vi "rsscope_core_global.vi"() -> ()   [LabVIEW 2014] (continued)
"Data Type"=0, "Command"="SEAR:TRIG:DPHY:ESDT:COND", "Access"=2, "Range Table"="rsscope_rngProtocolTriggerCondition", "Read Callback"="rsscope_FormatSearchNameInt32_ReadCallback.vi", "Write Callback"="rsscope_FormatSearchNameInt32_WriteCallback.vi", "Supported Models"="", "Instrument Options"="K42", "Flags"=0, "Help"="Set the condition for the escape mode data value. You can define an exact value or a value range.\n\nAvailable Repeated Capabilities:\nNone\n\nRemote-control command(s):\nSEARch:TRIGger:DPHY:ESDTa:CONDition"}, {"Level"=5, "Class Only"=FALSE, "Identifier"="RSSCOPE_ATTR_DPHY_SEARCH_LOW_POWER_ESCAPE_MODE_DATA_MIN", "Descriptive Name"="DPHY Search Low Power Escape Mode Data Min", "Data Type"=2, "Command"="SEAR:TRIG:DPHY:ESDT:MIN", "Access"=2, "Range Table"="", "Read Callback"="rsscope_FormatSearchNameString_ReadCallback.vi", "Write Callback"="rsscope_FormatSearchNameString_WriteCallback.vi", "Supported Models"="", "Instrument Options"="K42", "Flags"=0, "Help"="Specifies an escape mode data bit pattern, or sets the start value of a pattern range.\n\nValid Values:\nBinary pattern string consisting of 1; 0; or X (any bit).\n\nAvailable Repeated Capabilities:\nNone\n\nRemote-control command(s):\nSEARch:TRIGger:DPHY:ESDTa:MIN"}, {"Level"=5, "Class Only"=FALSE, "Identifier"="RSSCOPE_ATTR_DPHY_SEARCH_LOW_POWER_ESCAPE_MODE_DATA_MAX", "Descriptive Name"="DPHY Search Low Power Escape Mode Data Max", "Data Type"=2, "Command"="SEAR:TRIG:DPHY:ESDT:MAX", "Access"=2, "Range Table"="", "Read Callback"="rsscope_FormatSearchNameString_ReadCallback.vi", "Write Callback"="rsscope_FormatSearchNameString_WriteCallback.vi", "Supported Models"="", "Instrument Options"="K42", "Flags"=0, "Help"="Sets the end value of a escape mode data type range for condition In Range or Out of Range. \n\nValid Values:\nBinary pattern string consisting of 1; 0; or X (any bit).\n\nAvailable Repeated Capabilities:\nNone\n\nRemote-control command(s):\nSEARch:TRIGger:DPHY:ESDTa:MAX"}, {"Level"=4, "Class Only"=TRUE, "Identifier"="", "Descriptive Name"="Data Index", "Data Type"=0, "Command"="", "Access"=0, "Range Table"="", "Read Callback"="", "Write Callback"="", "Supported Models"="", "Instrument Options"="", "Flags"=0, "Help"="Data index sets the range within this series of the data value that is considered for the analysis. The data index setup consists of the condition and one or two data index values."}, {"Level"=5, "Class Only"=FALSE, "Identifier"="RSSCOPE_ATTR_DPHY_SEARCH_HIGH_SPEED_DATA_INDEX_CONDITION", "Descriptive Name"="DPHY Search High Speed Data Index Condition", "Data Type"=0, "Command"="SEAR:TRIG:DPHY:DIDX:COND", "Access"=2, "Range Table"="rsscope_rngProtocolTriggerCondition", "Read Callback"="rsscope_FormatSearchNameInt32_ReadCallback.vi", "Write Callback"="rsscope_FormatSearchNameInt32_WriteCallback.vi", "Supported Models"="", "Instrument Options"="K42", "Flags"=0, "Help"="Sets the condition for the data index. You can define an exact value or a value range.\n\nAvailable Repeated Capabilities:\nNone\n\nRemote-control command(s):\nSEARch:TRIGger:DPHY:DIDX:CONDition"}, {"Level"=5, "Class Only"=FALSE, "Identifier"="RSSCOPE_ATTR_DPHY_SEARCH_HIGH_SPEED_DATA_INDEX_MIN", "Descriptive Name"="DPHY Search High Speed Data Index Min", "Data Type"=0, "Command"="SEAR:TRIG:DPHY:DIDX:MIN", "Access"=2, "Range Table"="", "Read Callback"="rsscope_FormatSearchNameInt32_ReadCallback.vi", "Write Callback"="rsscope_FormatSearchNameInt32_WriteCallback.vi", "Supported Models"="", "Instrument Options"="K42", "Flags"=0, "Help"="Specifies a data index minimum, or sets the start value of a range.\n\nAvailable Repeated Capabilities:\nNone\n\nRemote-control command(s):\nSEARch:TRIGger:DPHY:DIDX:MIN"}, {"Level"=5, "Class Only"=FALSE, "Identifier"="RSSCOPE_ATTR_DPHY_SEARCH_HIGH_SPEED_DATA_INDEX_MAX", "Descriptive Name"="DPHY Search High Speed Data Index Max", "Data Type"=0, "Command"="SEAR:TRIG:DPHY:DIDX:MAX", "Access"=2, "Range Table"="", "Read Callback"="rsscope_FormatSearchNameInt32_ReadCallback.vi", "Write Callback"="rsscope_FormatSearchNameInt32_WriteCallback.vi", "Supported Models"="", "Instrument Options"="K42", "Flags"=0, "Help"="Sets the end value of a data index range for condition In Range or Out of Range.\n\nAvailable Repeated Capabilities:\nNone\n\nRemote-control command(s):\nSEARch:TRIGger:DPHY:DIDX:MAX"}, {"Level"=5, "Class Only"=FALSE, "Identifier"="RSSCOPE_ATTR_DPHY_SEARCH_LOW_POWER_ESCAPE_MODE_DATA_INDEX_CONDITION", "Descriptive Name"="DPHY Search Low Power Escape Mode Data Index Condition", "Data Type"=0, "Command"="SEAR:TRIG:DPHY:ESIN:COND", "Access"=2, "Range Table"="rsscope_rngProtocolTriggerCondition", "Read Callback"="rsscope_FormatSearchNameInt32_ReadCallback.vi", "Write Callback"="rsscope_FormatSearchNameInt32_WriteCallback.vi", "Supported Models"="", "Instrument Options"="K42", "Flags"=0, "Help"="Sets the condition for the escape mode data index. You can define an exact value or a value range.\n\nAvailable Repeated Capabilities:\nNone\n\nRemote-control command(s):\nSEARch:TRIGger:DPHY:ESINdex:CONDition"}, {"Level"=5, "Class Only"=FALSE, "Identifier"="RSSCOPE_ATTR_DPHY_SEARCH_LOW_POWER_ESCAPE_MODE_DATA_INDEX_MIN", "Descriptive Name"="DPHY Search Low Power Escape Mode Data Index Min", "Data Type"=0, "Command"="SEAR:TRIG:DPHY:ESIN:MIN", "Access"=2, "Range Table"="", "Read Callback"="rsscope_FormatSearchNameInt32_ReadCallback.vi", "Write Callback"="rsscope_FormatSearchNameInt32_WriteCallback.vi", "Supported Models"="", "Instrument Options"="K42", "Flags"=0, "Help"="Specifies an escape mode data index minimum, or sets the start value of a range.\n\nAvailable Repeated Capabilities:\nNone\n\nRemote-control command(s):\nSEARch:TRIGger:DPHY:ESINdex:MIN"}, {"Level"=5, "Class Only"=FALSE, "Identifier"="RSSCOPE_ATTR_DPHY_SEARCH_LOW_POWER_ESCAPE_MODE_DATA_INDEX_MAX", "Descriptive Name"="DPHY Search Low Power Escape Mode Data Index Max", "Data Type"=0, "Command"="SEAR:TRIG:DPHY:ESIN:MAX", "Access"=2, "Range Table"="", "Read Callback"="rsscope_FormatSearchNameInt32_ReadCallback.vi", "Write Callback"="rsscope_FormatSearchNameInt32_WriteCallback.vi", "Supported Models"="", "Instrument Options"="K42", "Flags"=0, "Help"="Sets the end value of a data index range for condition In Range or Out of Range.\n\nAvailable Repeated Capabilities:\nNone\n\nRemote-control command(s):\nSEARch:TRIGger:DPHY:ESINdex:MAX"}, {"Level"=4, "Class Only"=TRUE, "Identifier"="", "Descriptive Name"="Escape Mode", "Data Type"=0, "Command"="", "Access"=0, "Range Table"="", "Read Callback"="", "Write Callback"="", "Supported Models"="", "Instrument Options"="", "Flags"=0, "Help"="Set the specified data value to be searched for.The escape mode setup consists of the condition and one or two data patterns."}, {"Level"=5, "Class Only"=FALSE, "Identifier"="RSSCOPE_ATTR_DPHY_SEARCH_ESCAPE_MODE_CONDITION", "Descriptive Name"="DPHY Search Escape Mode Condition", "Data Type"=0, "Command"="SEAR:TRIG:DPHY:ESCM:COND", "Access"=2, "Range Table"="rsscope_rngProtocolTriggerCondition", "Read Callback"="rsscope_FormatSearchNameInt32_ReadCallback.vi", "Write Callback"="rsscope_FormatSearchNameInt32_WriteCallback.vi", "Supported Models"="", "Instrument Options"="K42", "Flags"=0, "Help"="Set the condition for the escape mode. You can define an exact value or a value range.\n\nAvailable Repeated Capabilities:\nNone\n\nRemote-control command(s):\nSEARch:TRIGger:DPHY:ESCMode:CONDition"}, {"Level"=5, "Class Only"=FALSE, "Identifier"="RSSCOPE_ATTR_DPHY_SEARCH_ESCAPE_MODE_MIN", "Descriptive Name"="DPHY Search Escape Mode Min", "Data Type"=2, "Command"="SEAR:TRIG:DPHY:ESCM:MIN", "Access"=2, "Range Table"="", "Read Callback"="rsscope_FormatSearchNameString_ReadCallback.vi", "Write Callback"="rsscope_FormatSearchNameString_WriteCallback.vi", "Supported Models"="", "Instrument Options"="K42", "Flags"=0, "Help"="Specifies a escape mode bit pattern, or sets the start value of a pattern range.\n\nValid Values:\nBinary pattern string consisting of 1; 0; or X (any bit).\n\nAvailable Repeated Capabilities:\nNone\n\nRemote-control command(s):\nSEARch:TRIGger:DPHY:ESCMode:MIN"}, {"Level"=5, "Class Only"=FALSE, "Identifier"="RSSCOPE_ATTR_DPHY_SEARCH_ESCAPE_MODE_MAX", "Descriptive Name"="DPHY Search Escape Mode Max", "Data Type"=2, "Command"="SEAR:TRIG:DPHY:ESCM:MAX", "Access"=2, "Range Table"="", "Read Callback"="rsscope_FormatSearchNameString_ReadCallback.vi", "Write Callback"="rsscope_FormatSearchNameString_WriteCallback.vi", "Supported Models"="", "Instrument Options"="K42", "Flags"=0, "Help"="Sets the end value of an escape mode range for condition In Range or Out of Range. \n\nValid Values:\nBinary pattern string consisting of 1; 0; or X (any bit).\n\nAvailable Repeated Capabilities:\nNone\n\nRemote-control command(s):\nSEARch:TRIGger:DPHY:ESCMode:MAX"}, {"Level"=4, "Class Only"=TRUE, "Identifier"="", "Descriptive Name"="Results", "Data Type"=0, "Command"="", "Access"=0, "Range Table"="", "Read Callback"="", "Write Callback"="", "Supported Models"="", "Instrument Options"="", "Flags"=0, "Help"="Returns the D-PHY search results."}, {"Level"=5, "Class Only"=FALSE, "Identifier"="RSSCOPE_ATTR_SEARCH_DPHY_FRAME_COUNT", "Descriptive Name"="Search DPHY Frame Count", "Data Type"=0, "Command"="SEAR:RES:DPHY:FCO?", "Access"=0, "Range Table"="", "Read Callback"="rsscope_FormatSearchNameInt32_ReadCallback.vi", "Write Callback"="", "Supported Models"="", "Instrument Options"="K42", "Flags"=0, "Help"="Returns the number of decoded frames for the selected serial bus.\n\nAvailable Repeated Capabilities:\nNone\n\nRemote-control command(s):\nSEARch:RESult:DPHY:FCOunt?"}, {"Level"=3, "Class Only"=TRUE, "Identifier"="", "Descriptive Name"="Space Wire", "Data Type"=0, "Command"="", "Access"=0, "Range Table"="", "Read Callback"="", "Write Callback"="", "Supported Models"="", "Instrument Options"="", "Flags"=0, "Help"="Configures Space Wire search."}, {"Level"=4, "Class Only"=FALSE, "Identifier"="RSSCOPE_ATTR_SPACE_WIRE_SEARCH_TYPE", "Descriptive Name"="Space Wire Search Type", "Data Type"=0, "Command"="SEAR:TRIG:SWIR:TYPE", "Access"=2, "Range Table"="RsScope_rngSpaceWireTriggerType", "Read Callback"="rsscope_FormatSearchNameInt32_ReadCallback.vi", "Write Callback"="rsscope_FormatSearchNameInt32_WriteCallback.vi", "Supported Models"="", "Instrument Options"="K65", "Flags"=0, "Help"="Sets the search type for the Space Wire analysis.\n\nAvailable Repeated Capabilities:\nNone\n\nRemote-control command(s):\nSEARch:TRIGger:SWIRe:TYPE"}, {"Level"=4, "Class Only"=FALSE, "Identifier"="RSSCOPE_ATTR_SPACE_WIRE_SEARCH_CONTROL_TYPE", "Descriptive Name"="Space Wire Search Control Type", "Data Type"=0, "Command"="SEAR:TRIG:SWIR:CTYP", "Access"=2, "Range Table"="RsScope_rngSpaceWireTriggerControlType", "Read Callback"="rsscope_FormatSearchNameInt32_ReadCallback.vi", "Write Callback"="rsscope_FormatSearchNameInt32_WriteCallback.vi", "Supported Models"="", "Instrument Options"="K65", "Flags"=0, "Help"="Searches for a specific control type character.\n\nAvailable Repeated Capabilities:\nNone\n\nRemote-control command(s):\nSEARch:TRIGger:SWIRe:CTYPe"}, {"Level"=4, "Class Only"=TRUE, "Identifier"="", "Descriptive Name"="Time Code", "Data Type"=0, "Command"="", "Access"=0, "Range Table"="", "Read Callback"="", "Write Callback"="", "Supported Models"="", "Instrument Options"="", "Flags"=0, "Help"="Sets the specified data type for the time code to be searched for. The data type setup consists of the condition and one or two data patterns."}, {"Level"=5, "Class Only"=FALSE, "Identifier"="RSSCOPE_ATTR_SPACE_WIRE_SEARCH_TIME_CODE_CONDITION", "Descriptive Name"="Space Wire Search Time Code Condition", "Data Type"=0, "Command"="SEAR:TRIG:SWIR:TIME:COND", "Access"=2, "Range Table"="rsscope_rngProtocolTriggerCondition", "Read Callback"="rsscope_FormatSearchNameInt32_ReadCallback.vi", "Write Callback"="rsscope_FormatSearchNameInt32_WriteCallback.vi", "Supported Models"="", "Instrument Options"="K65", "Flags"=0, "Help"="Set the condition for the data value for the time code. You can define an exact value or a value range.\n\nAvailable Repeated Capabilities:\nNone\n\nRemote-control command(s):\nSEARch:TRIGger:SWIRe:TIME:CONDition"}, {"Level"=5, "Class Only"=FALSE, "Identifier"="RSSCOPE_ATTR_SPACE_WIRE_SEARCH_TIME_CODE_MIN", "Descriptive Name"="Space Wire Search Time Code Min", "Data Type"=2, "Command"="SEAR:TRIG:SWIR:TIME:MIN", "Access"=2, "Range Table"="", "Read Callback"="rsscope_FormatSearchNameString_ReadCallback.vi", "Write Callback"="rsscope_FormatSearchNameString_WriteCallback.vi", "Supported Models"="", "Instrument Options"="K65", "Flags"=0, "Help"="Specifies a pattern for the data value for the time code, or sets the start value of a pattern range.\n\nValid Values:\nBinary pattern string consisting of 1; 0; or X (any bit).\n\nAvailable Repeated Capabilities:\nNone\n\nRemote-control command(s):\nSEARch:TRIGger:SWIRe:TIME:MIN"}, {"Level"=5, "Class Only"=FALSE, "Identifier"="RSSCOPE_ATTR_SPACE_WIRE_SEARCH_TIME_CODE_MAX", "Descriptive Name"="Space Wire Search Time Code Max", "Data Type"=2, "Command"="SEAR:TRIG:SWIR:TIME:MAX", "Access"=2, "Range Table"="", "Read Callback"="rsscope_FormatSearchNameString_ReadCallback.vi", "Write Callback"="rsscope_FormatSearchNameString_WriteCallback.vi", "Supported Models"="", "Instrument Options"="K65", "Flags"=0, "Help"="Sets the end value of a data value for the time code range for condition In Range or Out of Range. \n\nValid Values:\nBinary pattern string consisting of 1; 0; or X (any bit).\n\nAvailable Repeated Capabilities:\nNone\n\nRemote-control command(s):\nSEARch:TRIGger:SWIRe:TIME:MAX"}, {"Level"=4, "Class Only"=TRUE, "Identifier"="", "Descriptive Name"="Data", "Data Type"=0, "Command"="", "Access"=0, "Range Table"="", "Read Callback"="", "Write Callback"="", "Supported Models"="", "Instrument Options"="", "Flags"=0, "Help"="Sets the specified data type for the data pattern to be searched for. The data type setup consists of the condition and one or two data patterns."}, {"Level"=5, "Class Only"=FALSE, "Identifier"="RSSCOPE_ATTR_SPACE_WIRE_SEARCH_DATA_CONDITION", "Descriptive Name"="Space Wire Search Data Condition", "Data Type"=0, "Command"="SEAR:TRIG:SWIR:DATA:COND", "Access"=2, "Range Table"="rsscope_rngProtocolTriggerCondition", "Read Callback"="rsscope_FormatSearchNameInt32_ReadCallback.vi", "Write Callback"="rsscope_FormatSearchNameInt32_WriteCallback.vi", "Supported Models"="", "Instrument Options"="K65", "Flags"=0, "Help"="Set the condition for the data value. You can define an exact value or a value range.\n\nAvailable Repeated Capabilities:\nNone\n\nRemote-control command(s):\nSEARch:TRIGger:SWIRe:DATA:CONDition"}, {"Level"=5, "Class Only"=FALSE, "Identifier"="RSSCOPE_ATTR_SPACE_WIRE_SEARCH_DATA_MIN", "Descriptive Name"="Space Wire Search Data Min", "Data Type"=2, "Command"="SEAR:TRIG:SWIR:DATA:MIN", "Access"=2, "Range Table"="", "Read Callback"="rsscope_FormatSearchNameString_ReadCallback.vi", "Write Callback"="rsscope_FormatSearchNameString_WriteCallback.vi", "Supported Models"="", "Instrument Options"="K65", "Flags"=0, "Help"="Specifies a data for the data pattern, or sets the start value of a pattern range.\n\nValid Values:\nBinary pattern string consisting of 1; 0; or X (any bit).\n\nAvailable Repeated Capabilities:\nNone\n\nRemote-control command(s):\nSEARch:TRIGger:SWIRe:DATA:MIN"}, {"Level"=5, "Class Only"=FALSE, "Identifier"="RSSCOPE_ATTR_SPACE_WIRE_SEARCH_DATA_MAX", "Descriptive Name"="Space Wire Search Data Max", "Data Type"=2, "Command"="SEAR:TRIG:SWIR:DATA:MAX", "Access"=2, "Range Table"="", "Read Callback"="rsscope_FormatSearchNameString_ReadCallback.vi", "Write Callback"="rsscope_FormatSearchNameString_WriteCallback.vi", "Supported Models"="", "Instrument Options"="K65", "Flags"=0, "Help"="Sets the end value of a data for the data pattern range for condition In Range or Out of Range. \n\nValid Values:\nBinary pattern string consisting of 1; 0; or X (any bit).\n\nAvailable Repeated Capabilities:\nNone\n\nRemote-control command(s):\nSEARch:TRIGger:SWIRe:DATA:MAX"}, {"Level"=4, "Class Only"=TRUE, "Identifier"="", "Descriptive Name"="Error", "Data Type"=0, "Command"="", "Access"=0, "Range Table"="", "Read Callback"="", "Write Callback"="", "Supported Models"="", "Instrument Options"="", "Flags"=0, "Help"="Searches for the error."}, {"Level"=5, "Class Only"=FALSE, "Identifier"="RSSCOPE_ATTR_SPACE_WIRE_SEARCH_PARITY_ERROR", "Descriptive Name"="Space Wire Search Parity Error", "Data Type"=3, "Command"="SEAR:TRIG:SWIR:ERR:PAR", "Access"=2, "Range Table"="", "Read Callback"="rsscope_FormatSearchNameBoolean_ReadCallback.vi", "Write Callback"="rsscope_FormatSearchNameBoolean_WriteCallback.vi", "Supported Models"="", "Instrument Options"="K65", "Flags"=0, "Help"="Enables searching for a parity error (even parity).\n\nAvailable Repeated Capabilities:\nNone\n\nRemote-control command(s):\nSEARch:TRIGger:SWIRe:ERRor:PARity"}, {"Level"=5, "Class Only"=FALSE, "Identifier"="RSSCOPE_ATTR_SPACE_WIRE_SEARCH_ESCAPE_ERROR", "Descriptive Name"="Space Wire Search Escape Error", "Data Type"=3, "Command"="SEAR:TRIG:SWIR:ERR:ESC", "Access"=2, "Range Table"="", "Read Callback"="rsscope_FormatSearchNameBoolean_ReadCallback.vi", "Write Callback"="rsscope_FormatSearchNameBoolean_WriteCallback.vi", "Supported Models"="", "Instrument Options"="K65", "Flags"=0, "Help"="Enables searching for an escape error.\n\nAvailable Repeated Capabilities:\nNone\n\nRemote-control command(s):\nSEARch:TRIGger:SWIRe:ERRor:ESC"}, {"Level"=4, "Class Only"=TRUE, "Identifier"="", "Descriptive Name"="Results", "Data Type"=0, "Command"="", "Access"=0, "Range Table"="", "Read Callback"="", "Write Callback"="", "Supported Models"="", "Instrument Options"="", "Flags"=0, "Help"="Returns the Space Wire search results."}, {"Level"=5, "Class Only"=FALSE, "Identifier"="RSSCOPE_ATTR_SEARCH_SPACE_WIRE_FRAME_COUNT", "Descriptive Name"="Search Space Wire Frame Count", "Data Type"=0, "Command"="SEAR:RES:SWIR:FCO?", "Access"=0, "Range Table"="", "Read Callback"="rsscope_FormatSearchNameInt32_ReadCallback.vi", "Write Callback"="", "Supported Models"="", "Instrument Options"="K65", "Flags"=0, "Help"="Returns the number of frames within the search result for the selected serial bus.\n\nAvailable Repeated Capabilities:\nNone\n\nRemote-control command(s):\nSEARch:RESult:SWIRe:FCOunt?"}, {"Level"=3, "Class Only"=TRUE, "Identifier"="", "Descriptive Name"="SPI", "Data Type"=0, "Command"="", "Access"=0, "Range Table"="", "Read Callback"="", "Write Callback"="", "Supported Models"="", "Instrument Options"="", "Flags"=0, "Help"="In search setup commands, you must specify the <SearchName> parameter. It is a string parameter that contains the search definition name. All commands are similar to SPI trigger commands."}, {"Level"=4, "Class Only"=FALSE, "Identifier"="RSSCOPE_ATTR_SEARCH_SPI_MODE", "Descriptive Name"="Search SPI Mode", "Data Type"=0, "Command"="SEAR:TRIG:SPI:MODE", "Access"=2, "Range Table"="rsscope_rngProtocolSPITriggerType", "Read Callback"="rsscope_FormatSearchNameInt32_ReadCallback.vi", "Write Callback"="rsscope_FormatSearchNameInt32_WriteCallback.vi", "Supported Models"="", "Instrument Options"="", "Flags"=0, "Help"="Sets the event to be searched for.\n\nAvailable Repeated Capabilities:\nNone\n\nRemote-control command(s):\nSEARch:TRIGger:SPI:MODE"}, {"Level"=4, "Class Only"=FALSE, "Identifier"="RSSCOPE_ATTR_SEARCH_SPI_DATA_OPERATOR", "Descriptive Name"="Search SPI Data Operator", "Data Type"=0, "Command"="SEAR:TRIG:SPI:FCON", "Access"=2, "Range Table"="RsScope_rngSearchTriggerSPIDataOperator", "Read Callback"="rsscope_FormatSearchNameInt32_ReadCallback.vi", "Write Callback"="rsscope_FormatSearchNameInt32_WriteCallback.vi", "Supported Models"="", "Instrument Options"="", "Flags"=0, "Help"="Selects the operator for the data pattern: equal or not equal.\n\nAvailable Repeated Capabilities:\nNone\n\nRemote-control command(s):\nSEARch:TRIGger:SPI:FCONdition"}, {"Level"=4, "Class Only"=FALSE, "Identifier"="RSSCOPE_ATTR_SEARCH_SPI_MISO_PATTERN", "Descriptive Name"="Search SPI MISO Pattern", "Data Type"=2, "Command"="SEAR:TRIG:SPI:MIS", "Access"=2, "Range Table"="", "Read Callback"="rsscope_FormatSearchNamePattern_ReadCallback.vi", "Write Callback"="rsscope_FormatSearchNamePattern_WriteCallback.vi", "Supported Models"="", "Instrument Options"="", "Flags"=0, "Help"="Specifies a data pattern for the MISO line as a hex number.\n\nAvailable Repeated Capabilities:\nNone\n\nRemote-control command(s):\nSEARch:TRIGger:SPI:MISopattern"}, {"Level"=4, "Class Only"=FALSE, "Identifier"="RSSCOPE_ATTR_SEARCH_SPI_MOSI_PATTERN", "Descriptive Name"="Search SPI MOSI Pattern", "Data Type"=2, "Command"="SEAR:TRIG:SPI:MOS", "Access"=2, "Range Table"="", "Read Callback"="rsscope_FormatSearchNamePattern_ReadCallback.vi", "Write Callback"="rsscope_FormatSearchNamePattern_WriteCallback.vi", "Supported Models"="", "Instrument Options"="", "Flags"=0, "Help"="Specifies a data pattern for the MOSI line, as a hex number.\n\nAvailable Repeated Capabilities:\nNone\n\nRemote-control command(s):\nSEARch:TRIGger:SPI:MOSipattern"}, {"Level"=4, "Class Only"=FALSE, "Identifier"="RSSCOPE_ATTR_SEARCH_SPI_DATA_POSITION_OPERATOR", "Descriptive Name"="Search SPI Data Position Operator", "Data Type"=0, "Command"="SEAR:TRIG:SPI:DPOP", "Access"=2, "Range Table"="RsScope_rngSearchTriggerSPIDataPositionOperator", "Read Callback"="rsscope_FormatSearchNameInt32_ReadCallback.vi", "Write Callback"="rsscope_FormatSearchNameInt32_WriteCallback.vi", "Supported Models"="", "Instrument Options"="", "Flags"=0, "Help"="Operator for the data position. You can define an exact position, a position range, or let the position undefined (ANY).\n\nAvailable Repeated Capabilities:\nNone\n\nRemote-control command(s):\nSEARch:TRIGger:SPI:DPOPerator"}, {"Level"=4, "Class Only"=FALSE, "Identifier"="RSSCOPE_ATTR_SEARCH_SPI_DATA_POSITION", "Descriptive Name"="Search SPI Data Position", "Data Type"=0, "Command"="SEAR:TRIG:SPI:DPOS", "Access"=2, "Range Table"="RsScope_rngSearchTriggerSPIDataPosition", "Read Callback"="rsscope_FormatSearchNameInt32_ReadCallback.vi", "Write Callback"="rsscope_FormatSearchNameInt32_WriteCallback.vi", "Supported Models"="", "Instrument Options"="", "Flags"=0, "Help"="Sets the number of bits or words before the first word of interest.\n\nAvailable Repeated Capabilities:\nNone\n\nRemote-control command(s):\nSEARch:TRIGger:SPI:DPOSition"}, {"Level"=4, "Class Only"=FALSE, "Identifier"="RSSCOPE_ATTR_SEARCH_SPI_DATA_ALIGNMENT", "Descriptive Name"="Search SPI Data Alignment", "Data Type"=0, "Command"="SEAR:TRIG:SPI:PAL", "Access"=2, "Range Table"="rsscope_rngProtocolSPIDataAlignment", "Read Callback"="rsscope_FormatSearchNameInt32_ReadCallback.vi", "Write Callback"="rsscope_FormatSearchNameInt32_WriteCallback.vi", "Supported Models"="", "Instrument Options"="", "Flags"=0, "Help"="Defines how the specified data pattern is searched.\n\nAvailable Repeated Capabilities:\nNone\n\nRemote-control command(s):\nSEARch:TRIGger:SPI:PALignmen"}, {"Level"=4, "Class Only"=FALSE, "Identifier"="RSSCOPE_ATTR_SEARCH_SPI_DATA_POSITION_TO", "Descriptive Name"="Search SPI Data Position To", "Data Type"=0, "Command"="SEAR:TRIG:SPI:DPTO", "Access"=2, "Range Table"="RsScope_rngSearchTriggerSPIDataPosition", "Read Callback"="rsscope_FormatSearchNameInt32_ReadCallback.vi", "Write Callback"="rsscope_FormatSearchNameInt32_WriteCallback.vi", "Supported Models"="", "Instrument Options"="", "Flags"=0, "Help"="Sets the end value of a data postion range.\n\nAvailable Repeated Capabilities:\nNone\n\nRemote-control command(s):\nSEARch:TRIGger:SPI:DPTO"}, {"Level"=4, "Class Only"=TRUE, "Identifier"="", "Descriptive Name"="Results", "Data Type"=0, "Command"="", "Access"=0, "Range Table"="", "Read Callback"="", "Write Callback"="", "Supported Models"="", "Instrument Options"="", "Flags"=0, "Help"="The search on decoded SPI data returns the same results as the queries for decode\nresults."}, {"Level"=3, "Class Only"=TRUE, "Identifier"="", "Descriptive Name"="M-PHY", "Data Type"=0, "Command"="", "Access"=0, "Range Table"="", "Read Callback"="", "Write Callback"="", "Supported Models"="", "Instrument Options"="", "Flags"=0, "Help"="Contains attributes for M-PHY search."}, {"Level"=4, "Class Only"=FALSE, "Identifier"="RSSCOPE_ATTR_SEARCH_MPHY_TYPE", "Descriptive Name"="Search MPHY Type", "Data Type"=0, "Command"="SEAR:TRIG:MPHY:TYPE", "Access"=2, "Range Table"="RsScope_rngTriggerMPHYType", "Read Callback"="rsscope_FormatSearchNameInt32_ReadCallback.vi", "Write Callback"="rsscope_FormatSearchNameInt32_WriteCallback.vi", "Supported Models"="", "Instrument Options"="K44", "Flags"=0, "Help"="Selects the type of frame to be searched for.\n\nAvailable Repeated Capabilities:\nNone\n\nRemote-control command(s):\nSEARch:TRIGger:MPHY:TYPE"}, {"Level"=4, "Class Only"=FALSE, "Identifier"="RSSCOPE_ATTR_SEARCH_MPHY_LCC_TYPE", "Descriptive Name"="Search MPHY LCC Type", "Data Type"=0, "Command"="SEAR:TRIG:MPHY:LCCT", "Access"=2, "Range Table"="RsScope_rngTrigerMPHYLCCType", "Read Callback"="rsscope_FormatSearchNameInt32_ReadCallback.vi", "Write Callback"="rsscope_FormatSearchNameInt32_WriteCallback.vi", "Supported Models"="", "Instrument Options"="K44", "Flags"=0, "Help"="Selects the type of LCC frame to be searched for.\n\nAvailable Repeated Capabilities:\nNone\n\nRemote-control command(s):\nSEARch:TRIGger:MPHY:LCCType"}, {"Level"=4, "Class Only"=FALSE, "Identifier"="RSSCOPE_ATTR_SEARCH_MPHY_WORD_ONE_CONDITION", "Descriptive Name"="Search MPHY Word One Condition", "Data Type"=0, "Command"="SEAR:TRIG:MPHY:LWON:COND", "Access"=2, "Range Table"="RsScope_rngMPHYWordCondition", "Read Callback"="rsscope_FormatSearchNameInt32_ReadCallback.vi", "Write Callback"="rsscope_FormatSearchNameInt32_WriteCallback.vi", "Supported Models"="", "Instrument Options"="K44", "Flags"=0, "Help"="Sets the condition for WORD 1. You can define an exact value or a value range.\n\nAvailable Repeated Capabilities:\nNone\n\nRemote-control command(s):\nSEARch:TRIGger:MPHY:LWONe:CONDition"}, {"Level"=4, "Class Only"=FALSE, "Identifier"="RSSCOPE_ATTR_SEARCH_MPHY_WORD_ONE_MIN", "Descriptive Name"="Search MPHY Word One Min", "Data Type"=2, "Command"="SEAR:TRIG:MPHY:LWON:MIN", "Access"=2, "Range Table"="", "Read Callback"="rsscope_FormatSearchNameString_ReadCallback.vi", "Write Callback"="rsscope_FormatSearchNameString_WriteCallback.vi", "Supported Models"="", "Instrument Options"="K44", "Flags"=0, "Help"="Specifies the WORD 1 pattern, or sets the start value of a pattern range.\n\nAvailable Repeated Capabilities:\nNone\n\nRemote-control command(s):\nSEARch:TRIGger:MPHY:LWONe:MIN"}, {"Level"=4, "Class Only"=FALSE, "Identifier"="RSSCOPE_ATTR_SEARCH_MPHY_WORD_ONE_MAX", "Descriptive Name"="Search MPHY Word One Max", "Data Type"=2, "Command"="SEAR:TRIG:MPHY:LWON:MAX", "Access"=2, "Range Table"="", "Read Callback"="rsscope_FormatSearchNameString_ReadCallback.vi", "Write Callback"="rsscope_FormatSearchNameString_WriteCallback.vi", "Supported Models"="", "Instrument Options"="K44", "Flags"=0, "Help"="Sets the end value of the WORD 1 range if SEARch:TRIGger:MPHY:LWONe:CONDition is set to In Range or Out Of Range.\n\nAvailable Repeated Capabilities:\nNone\n\nRemote-control command(s):\nSEARch:TRIGger:MPHY:LWONe:MAX"}, {"Level"=4, "Class Only"=FALSE, "Identifier"="RSSCOPE_ATTR_SEARCH_MPHY_WORD_TWO_CONDITION", "Descriptive Name"="Search MPHY Word Two Condition", "Data Type"=0, "Command"="SEAR:TRIG:MPHY:LWTW:COND", "Access"=2, "Range Table"="RsScope_rngMPHYWordCondition", "Read Callback"="rsscope_FormatSearchNameInt32_ReadCallback.vi", "Write Callback"="rsscope_FormatSearchNameInt32_WriteCallback.vi", "Supported Models"="", "Instrument Options"="K44", "Flags"=0, "Help"="Sets the condition for WORD 2. You can define an exact value or a value range.\n\nAvailable Repeated Capabilities:\nNone\n\nRemote-control command(s):\nSEARch:TRIGger:MPHY:LWTWo:CONDition"}, {"Level"=4, "Class Only"=FALSE, "Identifier"="RSSCOPE_ATTR_SEARCH_MPHY_WORD_TWO_MIN", "Descriptive Name"="Search MPHY Word Two Min", "Data Type"=2, "Command"="SEAR:TRIG:MPHY:LWTW:MIN", "Access"=2, "Range Table"="", "Read Callback"="rsscope_FormatSearchNameString_ReadCallback.vi", "Write Callback"="rsscope_FormatSearchNameString_WriteCallback.vi", "Supported Models"="", "Instrument Options"="K44", "Flags"=0, "Help"="Specifies the WORD 2 pattern, or sets the start value of a pattern range.\n\nAvailable Repeated Capabilities:\nNone\n\nRemote-control command(s):\nSEARch:TRIGger:MPHY:LWTWo:MIN"}, {"Level"=4, "Class Only"=FALSE, "Identifier"="RSSCOPE_ATTR_SEARCH_MPHY_WORD_TWO_MAX", "Descriptive Name"="Search MPHY Word Two Max", "Data Type"=2, "Command"="SEAR:TRIG:MPHY:LWTW:MAX", "Access"=2, "Range Table"="", "Read Callback"="rsscope_FormatSearchNameString_ReadCallback.vi", "Write Callback"="rsscope_FormatSearchNameString_WriteCallback.vi", "Supported Models"="", "Instrument Options"="K44", "Flags"=0, "Help"="Sets the end value of the WORD 2 range if SEARch:TRIGger:MPHY:LWTWo:CONDition is set to In Range or Out Of Range.\n\nAvailable Repeated Capabilities:\nNone\n\nRemote-control command(s):\nSEARch:TRIGger:MPHY:LWTWo:MAX"}, {"Level"=4, "Class Only"=FALSE, "Identifier"="RSSCOPE_ATTR_SEARCH_MPHY_WORD_THREE_CONDITION", "Descriptive Name"="Search MPHY Word Three Condition", "Data Type"=0, "Command"="SEAR:TRIG:MPHY:LWTH:COND", "Access"=2, "Range Table"="RsScope_rngMPHYWordCondition", "Read Callback"="rsscope_FormatSearchNameInt32_ReadCallback.vi", "Write Callback"="rsscope_FormatSearchNameInt32_WriteCallback.vi", "Supported Models"="", "Instrument Options"="K44", "Flags"=0, "Help"="Sets the condition for WORD 3. You can define an exact value or a value range.\n\nAvailable Repeated Capabilities:\nNone\n\nRemote-control command(s):\nSEARch:TRIGger:MPHY:LWTHree:CONDition"}, {"Level"=4, "Class Only"=FALSE, "Identifier"="RSSCOPE_ATTR_SEARCH_MPHY_WORD_THREE_MIN", "Descriptive Name"="Search MPHY Word Three Min", "Data Type"=2, "Command"="SEAR:TRIG:MPHY:LWTH:MIN", "Access"=2, "Range Table"="", "Read Callback"="rsscope_FormatSearchNameString_ReadCallback.vi", "Write Callback"="rsscope_FormatSearchNameString_WriteCallback.vi", "Supported Models"="", "Instrument Options"="K44", "Flags"=0, "Help"="Specifies the WORD 3 pattern, or sets the start value of a pattern range.\n\nAvailable Repeated Capabilities:\nNone\n\nRemote-control command(s):\nSEARch:TRIGger:MPHY:LWTHree:MIN"}, {"Level"=4, "Class Only"=FALSE, "Identifier"="RSSCOPE_ATTR_SEARCH_MPHY_WORD_THREE_MAX", "Descriptive Name"="Search MPHY Word Three Max", "Data Type"=2, "Command"="SEAR:TRIG:MPHY:LWTH:MAX", "Access"=2, "Range Table"="", "Read Callback"="rsscope_FormatSearchNameString_ReadCallback.vi", "Write Callback"="rsscope_FormatSearchNameString_WriteCallback.vi", "Supported Models"="", "Instrument Options"="K44", "Flags"=0, "Help"="Sets the end value of the WORD 3 range if SEARch:TRIGger:MPHY:LWTHree:CONDition is set to In Range or Out Of Range.\n\nAvailable Repeated Capabilities:\nNone\n\nRemote-control command(s):\nSEARch:TRIGger:MPHY:LWTHree:MAX"}, {"Level"=4, "Class Only"=FALSE, "Identifier"="RSSCOPE_ATTR_SEARCH_MPHY_WORD_FOUR_CONDITION", "Descriptive Name"="Search MPHY Word Four Condition", "Data Type"=0, "Command"="SEAR:TRIG:MPHY:LWF:COND", "Access"=2, "Range Table"="RsScope_rngMPHYWordCondition", "Read Callback"="rsscope_FormatSearchNameInt32_ReadCallback.vi", "Write Callback"="rsscope_FormatSearchNameInt32_WriteCallback.vi", "Supported Models"="", "Instrument Options"="K44", "Flags"=0, "Help"="Sets the condition for WORD 4. You can define an exact value or a value range.\n\nAvailable Repeated Capabilities:\nNone\n\nRemote-control command(s):\nSEARch:TRIGger:MPHY:LWFour:CONDition"}, {"Level"=4, "Class Only"=FALSE, "Identifier"="RSSCOPE_ATTR_SEARCH_MPHY_WORD_FOUR_MIN", "Descriptive Name"="Search MPHY Word Four Min", "Data Type"=2, "Command"="SEAR:TRIG:MPHY:LWF:MIN", "Access"=2, "Range Table"="", "Read Callback"="rsscope_FormatSearchNameString_ReadCallback.vi", "Write Callback"="rsscope_FormatSearchNameString_WriteCallback.vi", "Supported Models"="", "Instrument Options"="K44", "Flags"=0, "Help"="Specifies the WORD 4 pattern, or sets the start value of a pattern range.\n\nAvailable Repeated Capabilities:\nNone\n\nRemote-control command(s):\nSEARch:TRIGger:MPHY:LWFour:MIN"}, {"Level"=4, "Class Only"=FALSE, "Identifier"="RSSCOPE_ATTR_SEARCH_MPHY_WORD_FOUR_MAX", "Descriptive Name"="Search MPHY Word Four Max", "Data Type"=2, "Command"="SEAR:TRIG:MPHY:LWF:MAX", "Access"=2, "Range Table"="", "Read Callback"="rsscope_FormatSearchNameString_ReadCallback.vi", "Write Callback"="rsscope_FormatSearchNameString_WriteCallback.vi", "Supported Models"="", "Instrument Options"="K44", "Flags"=0, "Help"="Sets the end value of the WORD 4 range if SEARch:TRIGger:MPHY:LWFour:CONDition is set to In Range or Out Of Range.\n\nAvailable Repeated Capabilities:\nNone\n\nRemote-control command(s):\nSEARch:TRIGger:MPHY:LWFour:MAX"}, {"Level"=4, "Class Only"=FALSE, "Identifier"="RSSCOPE_ATTR_SEARCH_MPHY_TC_PATTERN", "Descriptive Name"="Search MPHY TC Pattern", "Data Type"=2, "Command"="SEAR:TRIG:MPHY:TC", "Access"=2, "Range Table"="", "Read Callback"="rsscope_FormatSearchNameString_ReadCallback.vi", "Write Callback"="rsscope_FormatSearchNameString_WriteCallback.vi", "Supported Models"="", "Instrument Options"="K44", "Flags"=0, "Help"="Specifies the TC bit pattern.\n\nAvailable Repeated Capabilities:\nNone\n\nRemote-control command(s):\nSEARch:TRIGger:MPHY:TC"}, {"Level"=4, "Class Only"=FALSE, "Identifier"="RSSCOPE_ATTR_SEARCH_MPHY_DATA_CONDITION", "Descriptive Name"="Search MPHY Data Condition", "Data Type"=0, "Command"="SEAR:TRIG:MPHY:DATA:DCON", "Access"=2, "Range Table"="RsScope_rngMPHYWordCondition", "Read Callback"="rsscope_FormatSearchNameInt32_ReadCallback.vi", "Write Callback"="rsscope_FormatSearchNameInt32_WriteCallback.vi", "Supported Models"="", "Instrument Options"="K44", "Flags"=0, "Help"="Sets the condition for the data. You can define an exact value or a value range.\n\nAvailable Repeated Capabilities:\nNone\n\nRemote-control command(s):\nSEARch:TRIGger:MPHY:DATA:DCONdition"}, {"Level"=4, "Class Only"=FALSE, "Identifier"="RSSCOPE_ATTR_SEARCH_MPHY_DATA_MIN", "Descriptive Name"="Search MPHY Data Min", "Data Type"=2, "Command"="SEAR:TRIG:MPHY:DATA:DMIN", "Access"=2, "Range Table"="", "Read Callback"="rsscope_FormatSearchNameString_ReadCallback.vi", "Write Callback"="rsscope_FormatSearchNameString_WriteCallback.vi", "Supported Models"="", "Instrument Options"="K44", "Flags"=0, "Help"="Specifies the data bit pattern, or sets the start value of a pattern range.\n\nAvailable Repeated Capabilities:\nNone\n\nRemote-control command(s):\nSEARch:TRIGger:MPHY:DATA:DMIN"}, {"Level"=4, "Class Only"=FALSE, "Identifier"="RSSCOPE_ATTR_SEARCH_MPHY_DATA_MAX", "Descriptive Name"="Search MPHY Data Max", "Data Type"=2, "Command"="SEAR:TRIG:MPHY:DATA:DMAX", "Access"=2, "Range Table"="", "Read Callback"="rsscope_FormatSearchNameString_ReadCallback.vi", "Write Callback"="rsscope_FormatSearchNameString_WriteCallback.vi", "Supported Models"="", "Instrument Options"="K44", "Flags"=0, "Help"="Sets the end value of the data range if SEARch:TRIGger:MPHY:DATA:DCONdition is set to In Range or Out Of Range.\n\nAvailable Repeated Capabilities:\nNone\n\nRemote-control command(s):\nSEARch:TRIGger:MPHY:DATA:DMAX"}, {"Level"=4, "Class Only"=FALSE, "Identifier"="RSSCOPE_ATTR_SEARCH_MPHY_INDEX_CONDITION", "Descriptive Name"="Search MPHY Index Condition", "Data Type"=0, "Command"="SEAR:TRIG:MPHY:DATA:ICON", "Access"=2, "Range Table"="RsScope_rngMPHYWordCondition", "Read Callback"="rsscope_FormatSearchNameInt32_ReadCallback.vi", "Write Callback"="rsscope_FormatSearchNameInt32_WriteCallback.vi", "Supported Models"="", "Instrument Options"="K44", "Flags"=0, "Help"="Sets the condition for the index. You can define an exact value or a value range.\n\nAvailable Repeated Capabilities:\nNone\n\nRemote-control command(s):\nSEARch:TRIGger:MPHY:DATA:ICONdition"}, {"Level"=4, "Class Only"=FALSE, "Identifier"="RSSCOPE_ATTR_SEARCH_MPHY_INDEX_MIN", "Descriptive Name"="Search MPHY Index Min", "Data Type"=0, "Command"="SEAR:TRIG:MPHY:DATA:IMIN", "Access"=2, "Range Table"="RsScope_rngMPHYTriggerIndex", "Read Callback"="rsscope_FormatSearchNameInt32_ReadCallback.vi", "Write Callback"="rsscope_FormatSearchNameInt32_WriteCallback.vi", "Supported Models"="", "Instrument Options"="K44", "Flags"=0, "Help"="Specifies the index minimum, or sets the start value of a range.\n\nAvailable Repeated Capabilities:\nNone\n\nRemote-control command(s):\nSEARch:TRIGger:MPHY:DATA:IMIN"}, {"Level"=4, "Class Only"=FALSE, "Identifier"="RSSCOPE_ATTR_SEARCH_MPHY_INDEX_MAX", "Descriptive Name"="Search MPHY Index Max", "Data Type"=0, "Command"="SEAR:TRIG:MPHY:DATA:IMAX", "Access"=2, "Range Table"="RsScope_rngMPHYTriggerIndex", "Read Callback"="rsscope_FormatSearchNameInt32_ReadCallback.vi", "Write Callback"="rsscope_FormatSearchNameInt32_WriteCallback.vi", "Supported Models"="", "Instrument Options"="K44", "Flags"=0, "Help"="Sets the end value of the index range if SEARch:TRIGger:MPHY:DATA:ICONdition is set to INRange or RANge.\n\nAvailable Repeated Capabilities:\nNone\n\nRemote-control command(s):\nSEARch:TRIGger:MPHY:DATA:IMAX"}, {"Level"=4, "Class Only"=FALSE, "Identifier"="RSSCOPE_ATTR_SEARCH_MPHY_FSN_CONDITION", "Descriptive Name"="Search MPHY FSN Condition", "Data Type"=0, "Command"="SEAR:TRIG:MPHY:FSN:COND", "Access"=2, "Range Table"="RsScope_rngMPHYWordCondition", "Read Callback"="rsscope_FormatSearchNameInt32_ReadCallback.vi", "Write Callback"="rsscope_FormatSearchNameInt32_WriteCallback.vi", "Supported Models"="", "Instrument Options"="K44", "Flags"=0, "Help"="Sets the condition for FSN. You can define an exact value or a value range.\n\nAvailable Repeated Capabilities:\nNone\n\nRemote-control command(s):\nSEARch:TRIGger:MPHY:FSNumber:CONDition"}, {"Level"=4, "Class Only"=FALSE, "Identifier"="RSSCOPE_ATTR_SEARCH_MPHY_FSN_MIN", "Descriptive Name"="Search MPHY FSN Min", "Data Type"=2, "Command"="SEAR:TRIG:MPHY:FSN:MIN", "Access"=2, "Range Table"="", "Read Callback"="rsscope_FormatSearchNameString_ReadCallback.vi", "Write Callback"="rsscope_FormatSearchNameString_WriteCallback.vi", "Supported Models"="", "Instrument Options"="K44", "Flags"=0, "Help"="Specifies the FSN bit pattern, or sets the start value of a pattern range.\n\nAvailable Repeated Capabilities:\nNone\n\nRemote-control command(s):\nSEARch:TRIGger:MPHY:FSNumber:MIN"}, {"Level"=4, "Class Only"=FALSE, "Identifier"="RSSCOPE_ATTR_SEARCH_MPHY_FSN_MAX", "Descriptive Name"="Search MPHY FSN Max", "Data Type"=2, "Command"="SEAR:TRIG:MPHY:FSN:MAX", "Access"=2, "Range Table"="", "Read Callback"="rsscope_FormatSearchNameString_ReadCallback.vi", "Write Callback"="rsscope_FormatSearchNameString_WriteCallback.vi", "Supported Models"="", "Instrument Options"="K44", "Flags"=0, "Help"="Sets the end value of the FSN range if SEARch:TRIGger:MPHY:FSNumber:CONDition is set to In Range or Out Of Range.\n\nAvailable Repeated Capabilities:\nNone\n\nRemote-control command(s):\nSEARch:TRIGger:MPHY:FSNumber:MAX"}, {"Level"=4, "Class Only"=FALSE, "Identifier"="RSSCOPE_ATTR_SEARCH_MPHY_CRC_CONDITION", "Descriptive Name"="Search MPHY CRC Condition", "Data Type"=0, "Command"="SEAR:TRIG:MPHY:CRC:COND", "Access"=2, "Range Table"="RsScope_rngMPHYWordCondition", "Read Callback"="rsscope_FormatSearchNameInt32_ReadCallback.vi", "Write Callback"="rsscope_FormatSearchNameInt32_WriteCallback.vi", "Supported Models"="", "Instrument Options"="K44", "Flags"=0, "Help"="Sets the condition for CRC. You can define an exact value or a value range.\n\nAvailable Repeated Capabilities:\nNone\n\nRemote-control command(s):\nSEARch:TRIGger:MPHY:CRC:CONDition"}, {"Level"=4, "Class Only"=FALSE, "Identifier"="RSSCOPE_ATTR_SEARCH_MPHY_CRC_MIN", "Descriptive Name"="Search MPHY CRC Min", "Data Type"=2, "Command"="SEAR:TRIG:MPHY:CRC:MIN", 
